vi "dashboard.vi"() -> ()   [LabVIEW 2022 SP3]
uses:
  <userlib>/pcanbasic/constants/PCAN Bitrates.ctl
  <userlib>/pcanbasic/constants/PCAN Devices.ctl
  <userlib>/PCANBasic/PCANBasic.lvlib
panel:
  out "Found?":bool
  in  "stop":bool
  out "error out":errorcluster
  out "MessageBuffer out":T1 {"ID" format="%1x"}
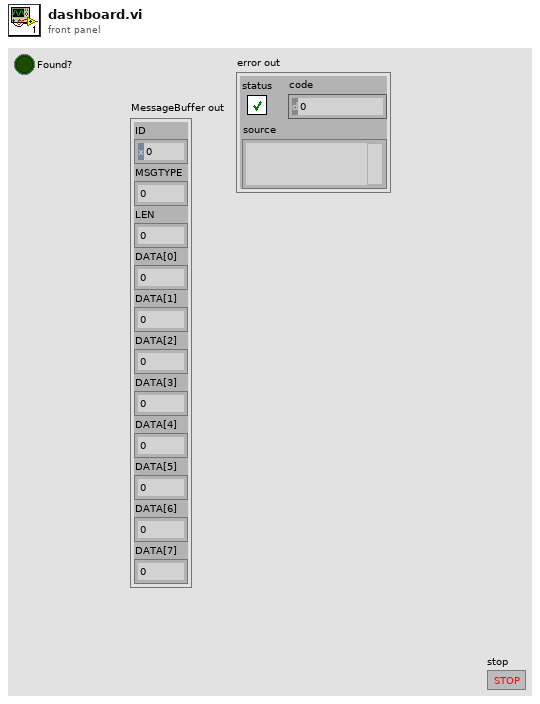
[diagram p1: front panel]
types:
  T1 = cluster{"ID":u32, "MSGTYPE":u8, "LEN":u8, "DATA[0]":u8, "DATA[1]":u8, "DATA[2]":u8, "DATA[3]":u8, "DATA[4]":u8, "DATA[5]":u8, "DATA[6]":u8, "DATA[7]":u8}
  T2 = typedef "PCANBasic.lvlib/PCAN Devices.ctl" = enum8{"PCAN_NONE", "PCAN_PEAKCAN", "PCAN_ISA", "PCAN_DNG", "PCAN_PCI", "PCAN_USB", "PCAN_PCC", "PCAN_VIRTUAL", "PCAN_LAN"}
  T3 = typedef "PCANBasic.lvlib/PCAN Bitrates.ctl" = u16
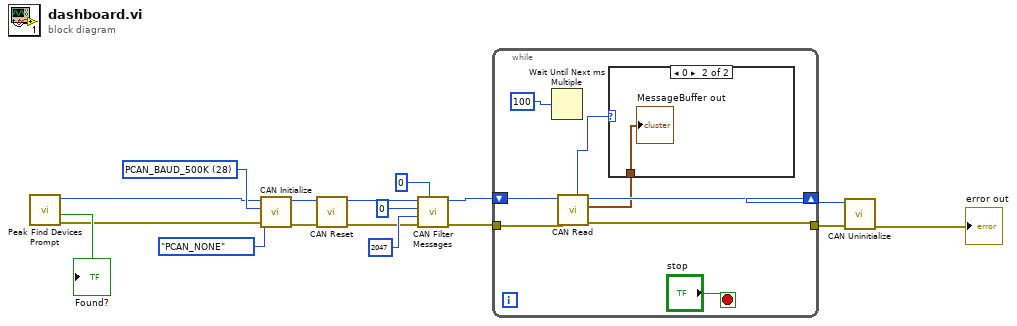
[diagram p0: block diagram]
diagram:
  w17 = T3 28 items=["PCAN_BAUD_1M"=20, "PCAN_BAUD_800K"=22, "PCAN_BAUD_500K"=28, "PCAN_BAUD_250K "=284, "PCAN_BAUD_125K "=796, "PCAN_BAUD_100K"=17199, "PCAN_BAUD_95K"=49998, "PCAN_BAUD_83K"=34091, "PCAN_BAUD_50K"=18223, "PCAN_BAUD_47K"=5140, "PCAN_BAUD_33K"=35631, "PCAN_BAUD_20K"=21295, "PCAN_BAUD_10K"=26415, "PCAN_BAUD_5K"=32639] ("PCAN Baud rate")
  n1 = call <userlib>:"Peak Find Devices Prompt.vi"() -> ("error out"=w2:errorcluster, "Found?"=→"Found?":bool, "CAN Channel"=w4:u16)  [unwired: 9 in]
  n2 = call <userlib>:"CAN Initialize.vi"("error in (no error)"=w2, "PCAN Devices"=PCAN_Devices."PCAN_NONE", "PCAN Baud rate"=w17, "Channel"=w4) -> ("error out"=w14:errorcluster, "Channel Out"=w15:u16)  [unwired: 5 in, 1 out]
  n3 = call <userlib>:"CAN Reset.vi"("error in (no error)"=w14, "Channel"=w15) -> ("error out"=w8:errorcluster, "Channel Out"=w11:u16)  [unwired: 7 in, 1 out]
  n4 = call <userlib>:"CAN Filter Messages.vi"("Mode"=u8 0, "error in (no error)"=w8, "ToID"=u32 2047, "FromID"=u32 0, "Channel"=w11) -> ("error out"=w6:errorcluster, "Channel Out"=w7:u16)  [unwired: 4 in, 1 out]
  n5 = while {
    shift-right: [w22] -> w1
    shift-left: w7 -> [w24]
    tunnel: w6 -> [w23]
    tunnel: [w25] -> w13
    stop <- "stop" stop-if-true
    n6 = Wait Until Next ms Multiple(millisecond multiple=u32 100) -> ()  [unwired: 1 out]
    n7 = call <userlib>:"CAN Read.vi"("error in (no error)"=w23, "Channel"=w24) -> ("error out"=w25:errorcluster, "MessageBuffer out"=w21:T1, "Channel Out"=w22:u16, "function return"=w18:u32)  [unwired: 5 in, 1 out]
    n8 = case shown="0" w18 {
      tunnel: w21 -> [_ w26]
      frame 1, Default {
      }
      frame 0 {
        "MessageBuffer out" <- w26
      }
    }
  }
  n9 = call <userlib>:"CAN Uninitialize.vi"("error in (no error)"=w13, "Channel"=w1) -> ("error out"=→"error out":errorcluster)  [unwired: 8 in, 1 out]
